vi "Online_Statistic_Read.vi"(8 "error in (no error)":errorcluster, 11 "Online_Statistic in":refnum<class "Online_Statistic.lvclass">) -> (0 "error out":errorcluster, 2 "stats_private":T1, 3 "Online_Statistic out":refnum<class "Online_Statistic.lvclass">)   [LabVIEW 2021, in "Online_Statistic.lvclass"]
uses:
  Online_Statistic.lvclass
  Online_Statistic.lvclass/Online_Statistic.ctl
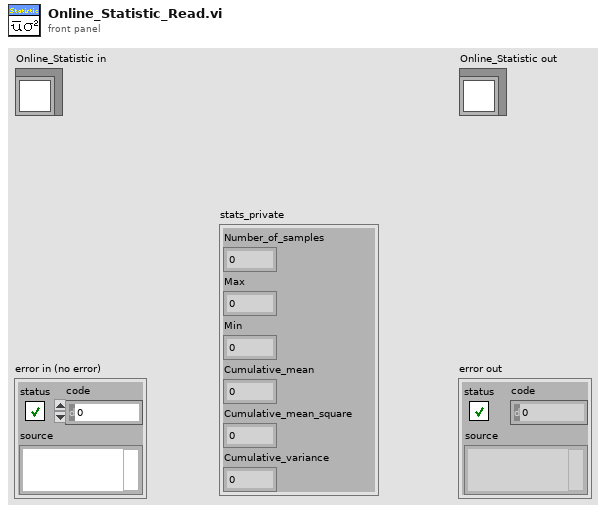
[diagram p1: front panel]
types:
  T1 = cluster{"Number_of_samples":i32, "Max":dbl, "Min":dbl, "Cumulative_mean":dbl, "Cumulative_mean_square ":dbl, "Cumulative_variance":dbl}
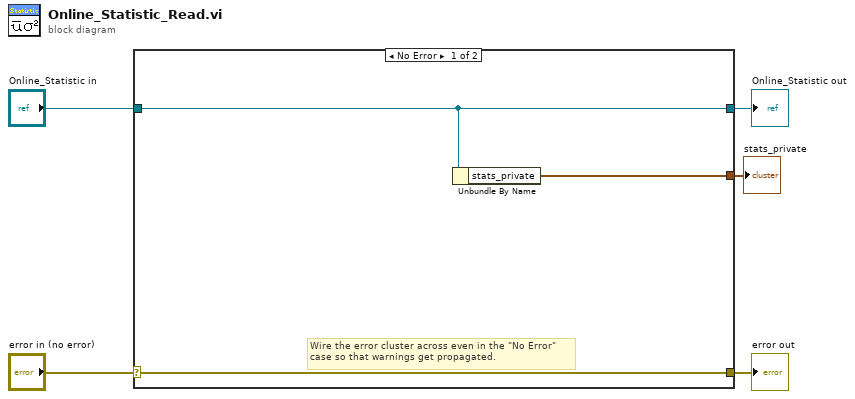
[diagram p0: block diagram]
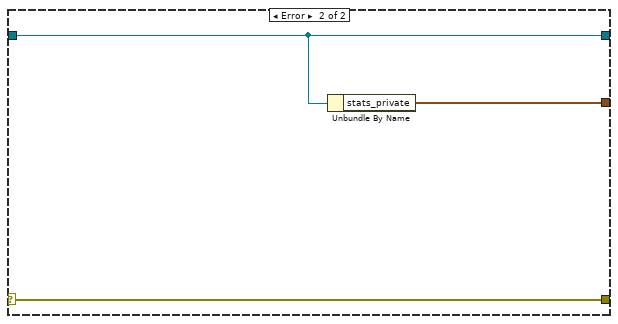
[diagram p2: hidden frame]
diagram:
  n1 = case shown="No Error" "error in (no error)" {
    selector: "error in (no error)" -> [w8 w11]
    tunnel: [w8 w11] -> w4
    tunnel: [w7 w10] -> w2
    tunnel: "Online_Statistic in" -> [w7 w10]
    tunnel: [w6 w9] -> w1
    frame No Error {
      # "Wire the error cluster across even in the \"No Error\"\ncase so that warnings get propagated."
      n2 = Unbundle By Name(w7) -> ("stats_private"=w6:T1)
    }
    frame Error {
      n3 = Unbundle By Name(w10) -> ("stats_private"=w9:T1)
    }
  }
  "error out" <- w4
  "Online_Statistic out" <- w2
  "stats_private" <- w1
